vi "InserExample.vi"   [LabVIEW 2017]
uses:
  <vilib>/addons/database/Connection.llb/DB Tools Open Connec (Path).vi
  <vilib>/addons/database/NI_Database_API.lvlib
types:
  T1 = typedef "NI_Database_API.lvlib/Conn ObjectReference.ctl" = refnum<k1>
  T2 = cluster{string, "date/time string":string, string, string, string, string}
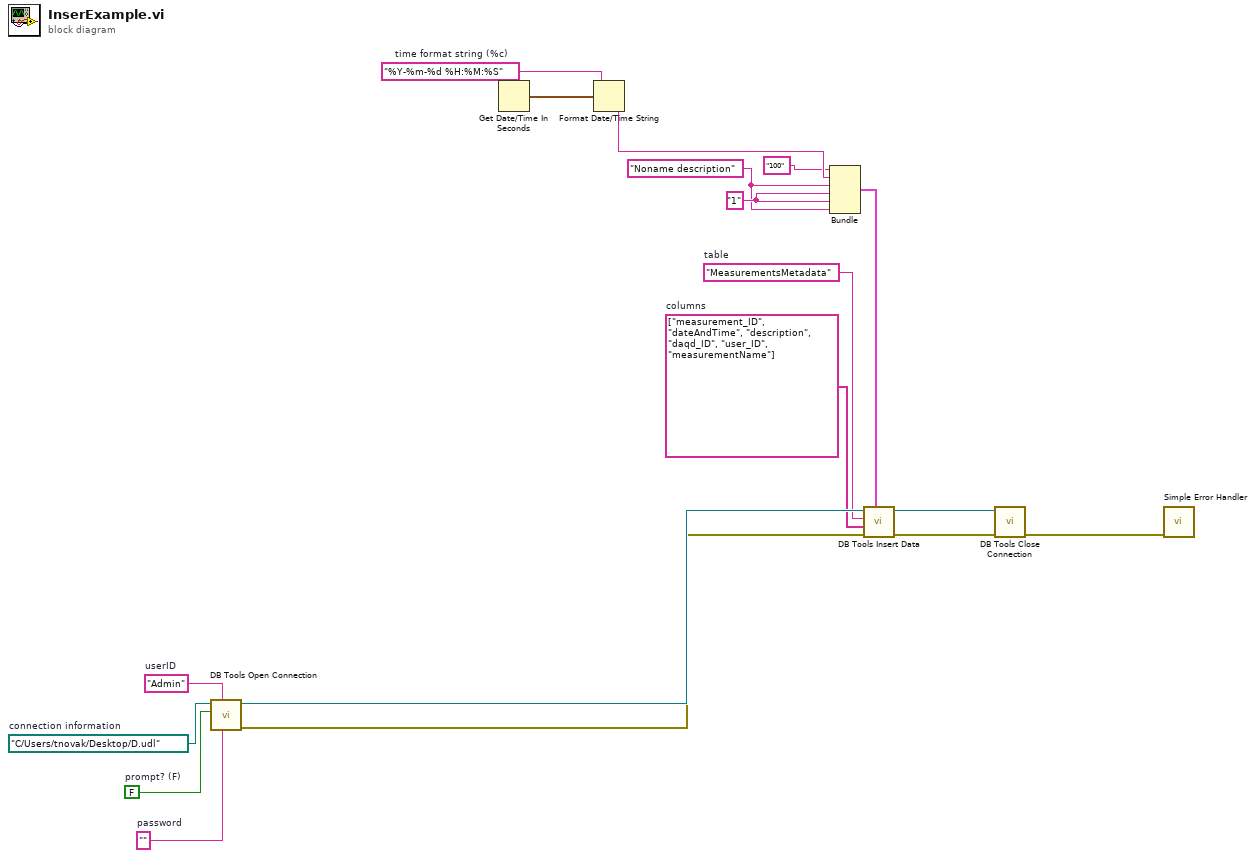
[diagram p0: block diagram]
diagram:
  w2 = "1"
  w1 = "Noname description"
  w6 = "MeasurementsMetadata"  # table
  w5 = string[] ["measurement_ID", "dateAndTime", "description", "daqd_ID", "user_ID", "measurementName"]  # columns
  w11 = path "C:/Users/tnovak/Desktop/D.udl"  # connection information
  w13 = ""  # password
  w14 = FALSE  # prompt? (F)
  w15 = "Admin"  # userID
  w17 = "%Y-%m-%d %H:%M:%S"  # time format string (%c)
  n1 = call-poly <vilib>:"DB Tools Open Connection.vi"("password"=w13, "userID"=w15, "prompt? (F)"=w14, "connection information"=w11) -> ("error out"=w9:errorcluster, "connection reference"=w10:T1)  [unwired: 4 in]
  n2 = Get Date/Time In Seconds() -> (seconds since 1Jan1904=w18:timestamp)
  n3 = Format Date/Time String(time format string (%c)=w17, seconds (now)=w18) -> (date/time string=w16:string)  [unwired: 1 in]
  n4 = Bundle("100", "date/time string"=w16, w1, w2, w2, w1) -> (w4:T2)  [unwired: 1 in]
  n5 = call <vilib>:"DB Tools Insert Data.vi"("data"=w4, "error in (no error)"=w9, "columns"=w5, "table"=w6, "connection reference"=w10) -> ("error out"=w8:errorcluster, "connection reference out"=w7:T1)  [unwired: 5 in]
  n6 = call <vilib>:"DB Tools Close Connection.vi"("error in (no error)"=w8, "connection reference"=w7) -> ("error out"=w12:errorcluster)  [unwired: 5 in]
  n7 = call <vilib>:"Simple Error Handler.vi"("error in (no error)"=w12) -> ()  [unwired: 4 in, 5 out]
